vi "Begin.vi"(8 "error in":errorcluster) -> (0 "error out":errorcluster)   [LabVIEW 2019]
doc: "Called before other user functions, this VI is expected to open initial I/O refnums, load in file data, and do all program initialization. Notice that the <B>error out</B> terminal is simply used for data flow. Wiring it to other structures or subVIs ensures that this VI runs first."
uses:
  <vilib>/Rock Robotics/SystemInterfaces/DIO/FPGA_DIOPWMChannel.ctl
  <vilib>/Rock Robotics/WPI/SafetyOutput/WPI_SafetyOutputConfigMenu.ctl
  <vilib>/Rock Robotics/WPI/DriverStation/WPI_DriverStationRobotMode2.ctl
  <vilib>/Rock Robotics/WPI/Joystick/WPI_JoystickDeviceEnum.ctl
  <vilib>/Rock Robotics/WPI/RobotDrive/WPI_RobotDriveOpen2MotorWithVictorSP.vi
  Robot Global Data.vi
  <vilib>/Rock Robotics/Network Tables/NT Write String Array.vi
  <vilib>/Rock Robotics/WPI/MotorControl/WPI_MotorControlOpen VictorSP.vi
  <vilib>/Rock Robotics/WPI/MotorControl/WPI_MotorControlOpen SPARK_MAX.vi
  <vilib>/Rock Robotics/WPI/MotorControl/WPI_MotorControlOpen TalonFX.vi
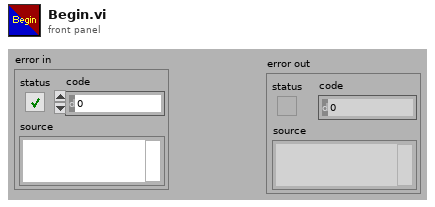
[diagram p1: front panel]
types:
  T1 = typedef "FPGA_DIOPWMChannel.ctl" = enum8{"PWM 0", "PWM 1", "PWM 2", "PWM 3", "PWM 4", "PWM 5", "PWM 6", "PWM 7", "PWM 8", "PWM 9", "PWM MXP 0", "PWM MXP 1", "PWM MXP 2", "PWM MXP 3", "PWM MXP 4", "PWM MXP 5", "PWM MXP 6", "PWM MXP 7", "PWM MXP 8", "PWM MXP 9", "Invalid"}
  T2 = typedef "WPI_JoystickDeviceEnum.ctl" = enum16{"USB 0", "USB 1", "USB 2", "USB 3", "USB 4", "USB 5"}
  T3 = typedef "WPI_DriverStationRobotMode2.ctl" = enum16{"Autonomous Disabled", "Autonomous Enabled", "Teleop Disabled", "Teleop Enabled", "Disconnected", "Finish", "Test Disabled", "Test Enabled", "Emergency Stopped"}
  T4 = typedef "WPI_SafetyOutputConfigMenu.ctl" = enum16{"Enable", "Disable"}
  T5 = typedef "WPI_RobotDriveDevRef.ctl" = cluster{"DevStatus":errorcluster, "Motors[]":T6[], "Square Inputs":bool, "Max Output":dbl}
  T6 = typedef "WPI_MotorControlDeviceRef.ctl" = cluster{"DeviceStatus":errorcluster, "Type":T7, "PWM":cluster{"PWM Channel":T1, "DeadBand":T8}, "CAN":cluster{"Device Number":u8, "SetOutput VI Ref":variant, "GetOutput VI Ref":variant, "Enable VI Ref":variant, "Disable VI Ref":variant, "Data":variant}, "Invert":bool, "DIO PWM":cluster{"PWM \"Enable\" Channel":T1, "DIOChannel":T9, "PWM Rate":dbl}}
  T7 = typedef "WPI_MotorControlType.ctl" = enum16{"PWM", "CAN", "DIO PWM"}
  T8 = typedef "WPI_PWMDeadband.ctl" = cluster{"Name":string, "maxPositivePwm":i32, "minPositivePwm":i32, "centerPwm":i32, "maxNegativePwm":i32, "minNegativePwm":i32, "angularRange":u16}
  T9 = typedef "FPGA_DIOChannel.ctl" = enum8{"DIO 0", "DIO 1", "DIO 2", "DIO 3", "DIO 4", "DIO 5", "DIO 6", "DIO 7", "DIO 8", "DIO 9", "DIO MXP 0", "DIO MXP 1", "DIO MXP 2", "DIO MXP 3", "DIO MXP 4", "DIO MXP 5", "DIO MXP 6", "DIO MXP 7", "DIO MXP 8", "DIO MXP 9", "DIO MXP 10", "DIO MXP 11", "DIO MXP 12", "DIO MXP 13", "DIO MXP 14", "DIO MXP 15", "SPI Port CS1", "SPI Port CS2", "SPI Port CS3", "SPI Port MISO", "SPI Port MOSI", "Invalid"}
  T10 = typedef "WPI_JoystickDevRef.ctl" = cluster{"Device":T2}
  T11 = typedef "WPI_ServoDeviceRef.ctl" = cluster{"DeviceStatus":errorcluster, "PWM Channel":T1, "DeadBand":T8}
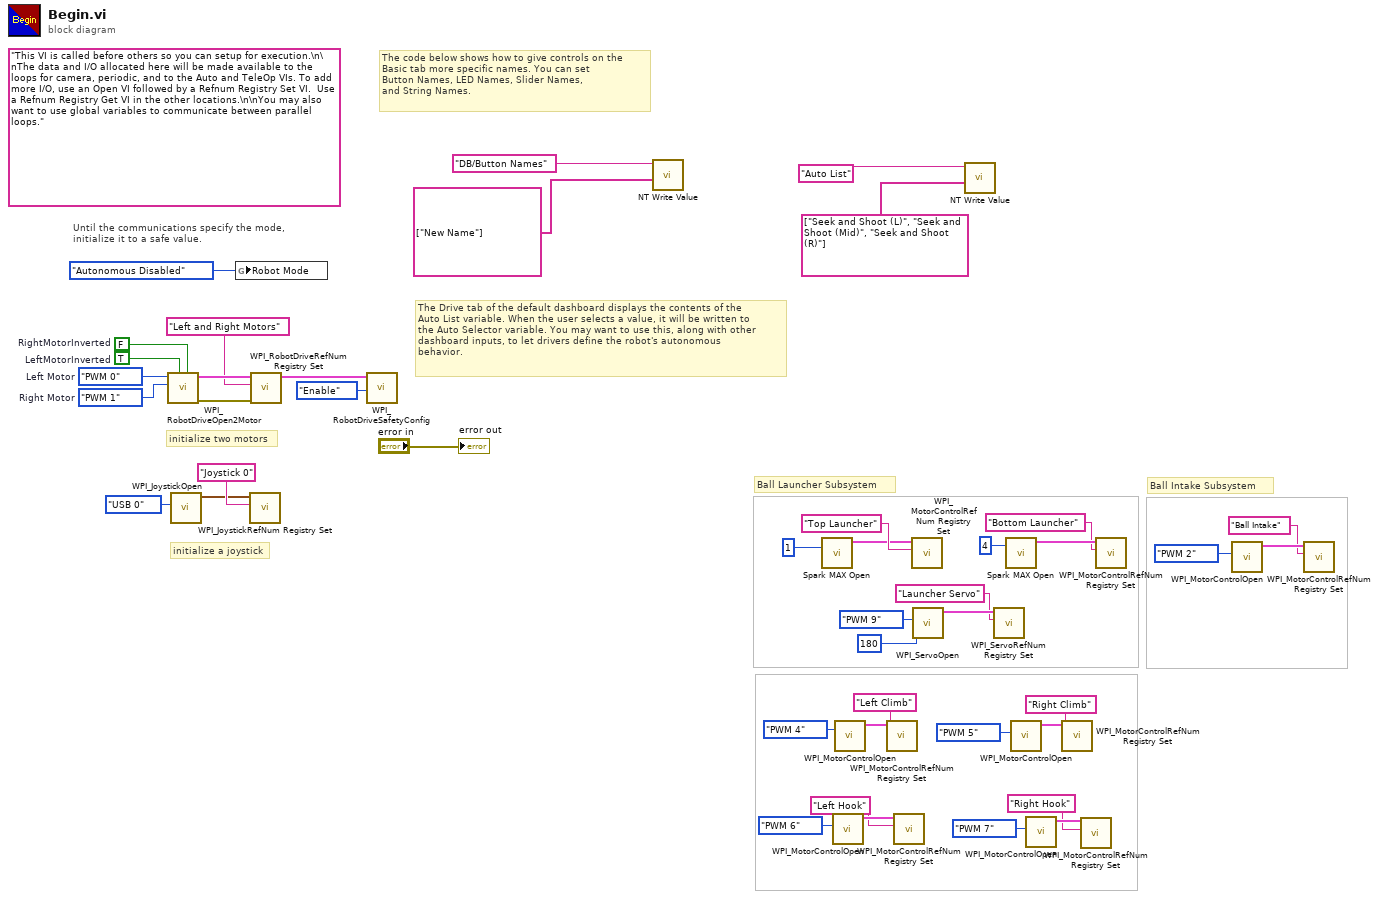
[diagram p0: block diagram]
diagram:
  (unwired) "This VI is called before others so you can setup for execution.\n\nThe data and I/O allocated here will be made available to the loops for camera, periodic, and to the Auto and TeleOp VIs. To add more I/O, use an Open VI followed by a Refnum Registry Set VI.  Use a Refnum Registry Get VI in the other locations.\n\nYou may also want to use global variables to communicate between parallel loops."
  w37 = FPGA_DIOPWMChannel."PWM 1"  # Right Motor
  w38 = FPGA_DIOPWMChannel."PWM 0"  # Left Motor
  w42 = TRUE  # LeftMotorInverted
  w43 = FALSE  # RightMotorInverted
  # "Ball Intake Subsystem"
  # "Ball Launcher Subsystem"
  # "The Drive tab of the default dashboard displays the contents of the\nAuto List variable. When the user selects a value, it will be written to\nthe Auto Selector variable. You may want to use this, along with other\ndashboard inputs, to let drivers define the robot's autonomous\nbehavior."
  # "The code below shows how to give controls on the\nBasic tab more specific names. You can set\nButton Names, LED Names, Slider Names,\nand String Names."
  # "initialize a joystick"
  # "Until the communications specify the mode,\ninitialize it to a safe value."
  # "initialize two motors"
  n1 = call-poly <vilib>:"WPI_RobotDriveOpen2Motor.vi"("Right Motor Inverted"=w43, "Left Motor Inverted"=w42, "Right Motor"=w37, "Left Motor"=w38) -> ("error out"=w39:errorcluster, "RobotDriveDevRef"=w41:T5)  [unwired: 1 in, 5 out]
  n2 = call <vilib>:"WPI_JoystickOpen.vi"("JoystickDevice"=WPI_JoystickDeviceEnum."USB 0") -> ("JoystickDevRef"=w32:T10)  [unwired: 10 in]
  n3 = global write "Robot Global Data.vi" "Robot Mode"(WPI_DriverStationRobotMode2."Autonomous Disabled" ("Robot Mode")) -> ()
  n4 = call <vilib>:"WPI_JoystickRefNum Registry Set.vi"("refnum name"="Joystick 0", "JoystickDevRef"=w32) -> ()  [unwired: 8 in, 2 out]
  n5 = call <vilib>:"WPI_RobotDriveRefNum Registry Set.vi"("error in (no error)"=w39, "refnum name"="Left and Right Motors", "RobotDriveDevRef"=w41) -> ("RobotDriveDevRef"=w36:T5)  [unwired: 1 in, 7 out]
  n6 = call <vilib>:"WPI_RobotDriveSafetyConfig.vi"("mode"=WPI_SafetyOutputConfigMenu."Enable", "RobotDriveDevRef"=w36) -> ()  [unwired: 8 in, 2 out]
  n7 = call-poly <vilib>:"NT Write Value.vi"("String Array"=string[] ["New Name"], "Name"="DB/Button Names") -> ()  [unwired: 9 in, 1 out]
  n8 = call <vilib>:"Spark MAX Open.vi"("Device Number"=u8 1) -> ("MotorControlDeviceRef"=w3:T6)  [unwired: 9 in, 1 out]
  n9 = call-poly <vilib>:"WPI_MotorControlOpen.vi"("PWM Channel"=FPGA_DIOPWMChannel."PWM 6") -> ("MotorControlDeviceRef"=w16:T6)  [unwired: 9 in, 1 out]
  n10 = call-poly <vilib>:"WPI_MotorControlOpen.vi"("PWM Channel"=FPGA_DIOPWMChannel."PWM 4") -> ("MotorControlDeviceRef"=w20:T6)  [unwired: 9 in, 1 out]
  n11 = call <vilib>:"WPI_MotorControlRefNum Registry Set.vi"("refnum name"="Left Climb", "MotorControlDevRef"=w20) -> ()  [unwired: 8 in, 2 out]
  n12 = call <vilib>:"WPI_MotorControlRefNum Registry Set.vi"("refnum name"="Left Hook", "MotorControlDevRef"=w16) -> ()  [unwired: 8 in, 2 out]
  n13 = call <vilib>:"WPI_MotorControlRefNum Registry Set.vi"("refnum name"="Top Launcher", "MotorControlDevRef"=w3) -> ()  [unwired: 8 in, 2 out]
  n14 = call <vilib>:"WPI_ServoOpen.vi"("Angular Range"=u16 180, "PWM Channel"=FPGA_DIOPWMChannel."PWM 9") -> ("ServoDeviceRef"=w9:T11)  [unwired: 8 in, 1 out]
  n15 = call-poly <vilib>:"NT Write Value.vi"("String Array"=string[] ["Seek and Shoot (L)", "Seek and Shoot (Mid)", "Seek and Shoot (R)"], "Name"="Auto List") -> ()  [unwired: 9 in, 1 out]
  n16 = call <vilib>:"WPI_ServoRefNum Registry Set.vi"("refnum name"="Launcher Servo", "ServoDeviceRef"=w9) -> ()  [unwired: 8 in, 2 out]
  n17 = call <vilib>:"Spark MAX Open.vi"("Device Number"=u8 4) -> ("MotorControlDeviceRef"=w2:T6)  [unwired: 9 in, 1 out]
  n18 = call-poly <vilib>:"WPI_MotorControlOpen.vi"("PWM Channel"=FPGA_DIOPWMChannel."PWM 5") -> ("MotorControlDeviceRef"=w18:T6)  [unwired: 9 in, 1 out]
  n19 = call-poly <vilib>:"WPI_MotorControlOpen.vi"("PWM Channel"=FPGA_DIOPWMChannel."PWM 7") -> ("MotorControlDeviceRef"=w15:T6)  [unwired: 9 in, 1 out]
  n20 = call <vilib>:"WPI_MotorControlRefNum Registry Set.vi"("refnum name"="Right Climb", "MotorControlDevRef"=w18) -> ()  [unwired: 8 in, 2 out]
  n21 = call <vilib>:"WPI_MotorControlRefNum Registry Set.vi"("refnum name"="Right Hook", "MotorControlDevRef"=w15) -> ()  [unwired: 8 in, 2 out]
  n22 = call <vilib>:"WPI_MotorControlRefNum Registry Set.vi"("refnum name"="Bottom Launcher", "MotorControlDevRef"=w2) -> ()  [unwired: 8 in, 2 out]
  n23 = call-poly <vilib>:"WPI_MotorControlOpen.vi"("PWM Channel"=FPGA_DIOPWMChannel."PWM 2") -> ("MotorControlDeviceRef"=w25:T6)  [unwired: 9 in, 1 out]
  n24 = call <vilib>:"WPI_MotorControlRefNum Registry Set.vi"("refnum name"="Ball Intake", "MotorControlDevRef"=w25) -> ()  [unwired: 8 in, 2 out]
  "error out" <- "error in"
